vi "SubMean.vi"(4 "Bit Depth":i32=8, 5 "Scan Data In":dbl[][](array[numeric]), 6 "Samp Rate (MHz)":i16, 7 "Filter Prams":T1={"low cutoff"=5, "order"=81, "high cutoff"=35}, 8 "Type of Mean":T2) -> (0 "Array":dbl[][](array[numeric]), 2 "Filter Params":T1, 3 "means":dbl[](array[numeric]))   [LabVIEW 2022 SP3]
uses:
  ViewData/-ReadEye/TypeDefs/TypeofMean.ctl
  <vilib>/Analysis/baseanly.llb/Mean (DBL).vi
  <vilib>/Analysis/2dsp.llb/1D Convolution (DBL).vi
  <vilib>/Analysis/NI_AALPro.lvlib
  <vilib>/Analysis/NI_AALBase.lvlib
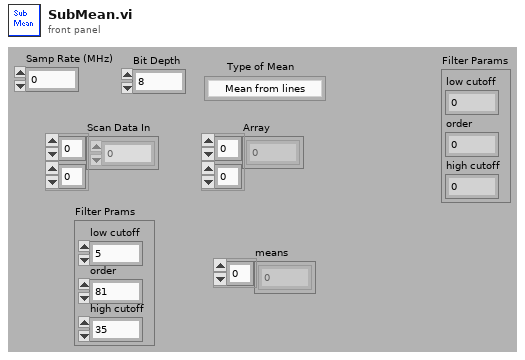
[diagram p1: front panel]
types:
  T1 = cluster{"low cutoff":i32, "order":i32, "high cutoff":i32}
  T2 = typedef "TypeofMean.ctl" = enum16{"Mean from lines", "Mean just lines", "Poly Mean", "No mean", "Filter"}
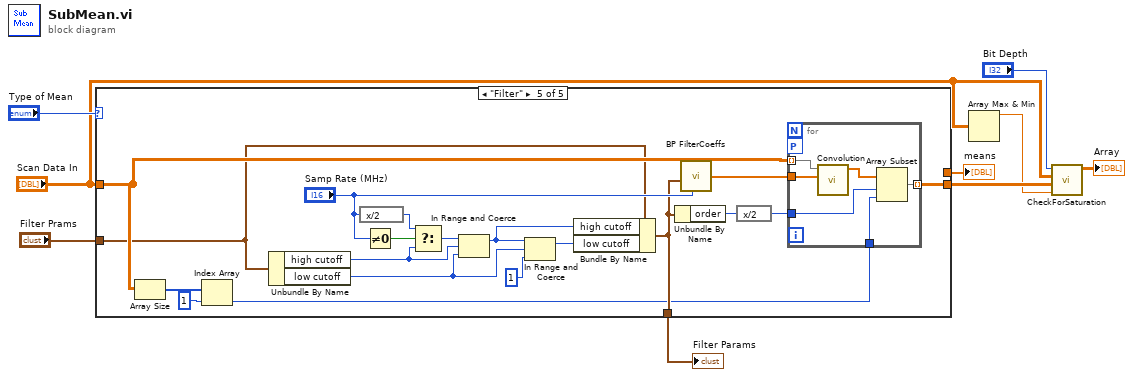
[diagram p0: block diagram]
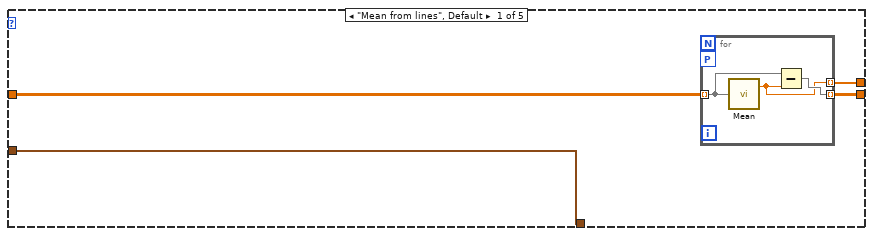
[diagram p2: hidden frame]
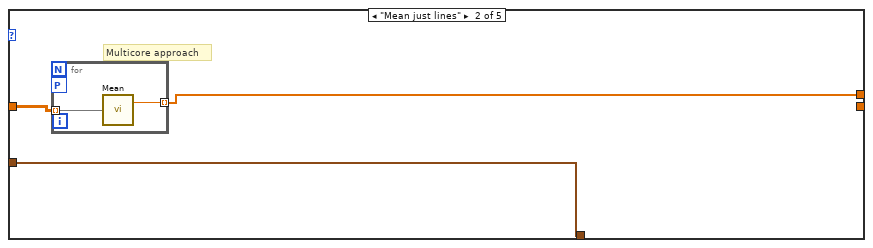
[diagram p3: hidden frame]
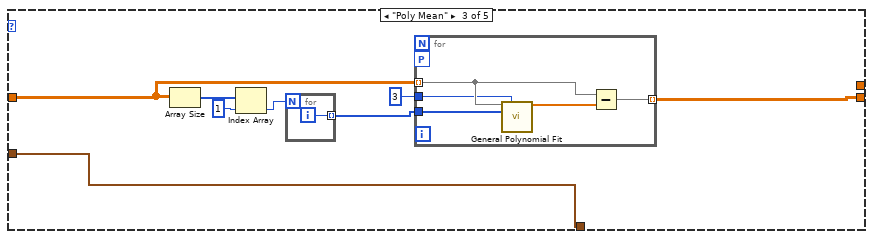
[diagram p4: hidden frame]
diagram:
  n1 = case shown="\"Filter\"" "Type of Mean" {
    tunnel: "Scan Data In" -> [w11 w19 w28 w37 w51]
    tunnel: [w12 _ w29 w37 w50] -> w4
    tunnel: [w13 w18 _ _ _] -> w9
    tunnel: "Filter Prams" -> [w10 w17 w22 w36 w40]
    tunnel: [w10 w17 w22 w36 w39] -> w6
    frame "Mean from lines", Default {
      n2 = for {
        tunnel: w11 -> [w16] mode=indexing
        tunnel: [w15] -> w12 mode=indexing
        tunnel: [w14] -> w13 mode=indexing
        workers-P: _ -> [_]
        n3 = call-poly <vilib>:"Mean.vi"("X"=w16) -> ("mean"=w14:dbl)  [unwired: 1 out]
        n4 = Subtract(x=w16, y=w14) -> (x-y=w15:dbl[])
      }
    }
    frame "Mean just lines" {
      # "Multicore approach"
      n5 = for {
        tunnel: w19 -> [w20] mode=indexing
        tunnel: [w21] -> w18 mode=indexing
        workers-P: _ -> [_]
        n6 = call-poly <vilib>:"Mean.vi"("X"=w20) -> ("mean"=w21:dbl)  [unwired: 1 out]
      }
    }
    frame "Poly Mean" {
      n7 = Array Size(array=w28) -> (size(s)=w27:i32[])
      n8 = Index Array(array=w27, index=1) -> (element=w26:i32)
      n9 = for {
        N: w26 -> [_]
        tunnel: [w30] -> w25 mode=indexing
        i -> [w30]
      }
      n10 = for {
        tunnel: w28 -> [w34] mode=indexing
        tunnel: [w33] -> w29 mode=indexing
        tunnel: w25 -> [w32]
        tunnel: 3 -> [w31]
        workers-P: _ -> [_]
        n11 = call <vilib>:"General Polynomial Fit.vi"("Y"=w34, "polynomial order"=w31, "X"=w32) -> ("Best Polynomial Fit"=w35:dbl[])  [unwired: 9 in, 3 out]
        n12 = Subtract(x=w34, y=w35) -> (x-y=w33:dbl[])
      }
    }
    frame "No mean" {
    }
    frame "Filter" {
      n13 = Array Size(array=w51) -> (size(s)=w54:i32[])
      n14 = Index Array(array=w54, index=1) -> (element=w38:i32)
      n15 = Unbundle By Name(w40) -> ("high cutoff"=w45:i32, "low cutoff"=w43:i32)
      n16 = expression code="x/2"("Samp Rate (MHz)") -> (w47:i16)
      n17 = Not Equal To 0?(x="Samp Rate (MHz)") -> (x != 0?=w48:bool)
      n18 = Select(t=w47, s=w48, f=w45) -> (s? t:f=w46:i32)
      n19 = In Range and Coerce(upper limit=w46, x=w45, lower limit=w43) -> (coerced(x)=w42:i32)  [unwired: 1 out]
      n20 = In Range and Coerce(upper limit=w42, x=w43, lower limit=1) -> (coerced(x)=w41:i32)  [unwired: 1 out]
      n21 = Bundle By Name(cluster=w40, "high cutoff"=w42, "low cutoff"=w41) -> (w39:T1)
      n22 = Unbundle By Name(w39) -> ("order"=w56:i32)
      n23 = call "BP FilterCoeffs.vi"("sample rate MHz"="Samp Rate (MHz)", "Filter Prams"=w39) -> ("FIR Windowed Coefficients"=w52:dbl[])  [unwired: 4 in]
      n24 = expression code="x/2"(w56) -> (w55:i32)
      n25 = for {
        tunnel: w55 -> [w58]
        tunnel: [w62] -> w50 mode=indexing
        tunnel: w51 -> [w61] mode=indexing
        workers-P: _ -> [_]
        tunnel: w52 -> [w60]
        tunnel: w38 -> [w57]
        n26 = call-poly <vilib>:"Convolution.vi"("Y"=w60, "X"=w61) -> ("X * Y"=w59:dbl[])  [unwired: 1 in, 8 out]
        n27 = Array Subset(array=w59, index=w58, length=w57) -> (w62:dbl[])
      }
    }
  }
  "means" <- w9
  "Filter Params" <- w6
  n28 = Array Max & Min(array="Scan Data In") -> (max value=w2:dbl)  [unwired: 3 out]
  n29 = call "CheckForSaturation.vi"("Replace Sat with X?"=w2, "Processed Data"=w4, "Original Data In"="Scan Data In", "Bit Depth"="Bit Depth") -> ("Data with Saturation"=→"Array":dbl[][])  [unwired: 7 in]
